vi "PathPlanner_PathFinder_DoReset.vi"   [LabVIEW 2019]
uses:
  PathPlannerLib24/VI/PathPlanner_GridPosition_Get.vi
  PathPlannerLib24/VI/PathPlanner_PathFinder_Heuristic.vi
  PathPlannerLib24/VI/PathPlanner_PathFinder_Globals.vi
  PathPlannerLib24/PathPlanner24.lvlib
types:
  T1 = typedef "PathPlanner24.lvlib/PathPlannerFinderGridPosition.ctl" = cluster{"X":i32, "Y":i32}
  T2 = typedef "PathPlanner24.lvlib/PathPlannerFinderDoublePair.ctl" = cluster{"A":dbl, "B":dbl}
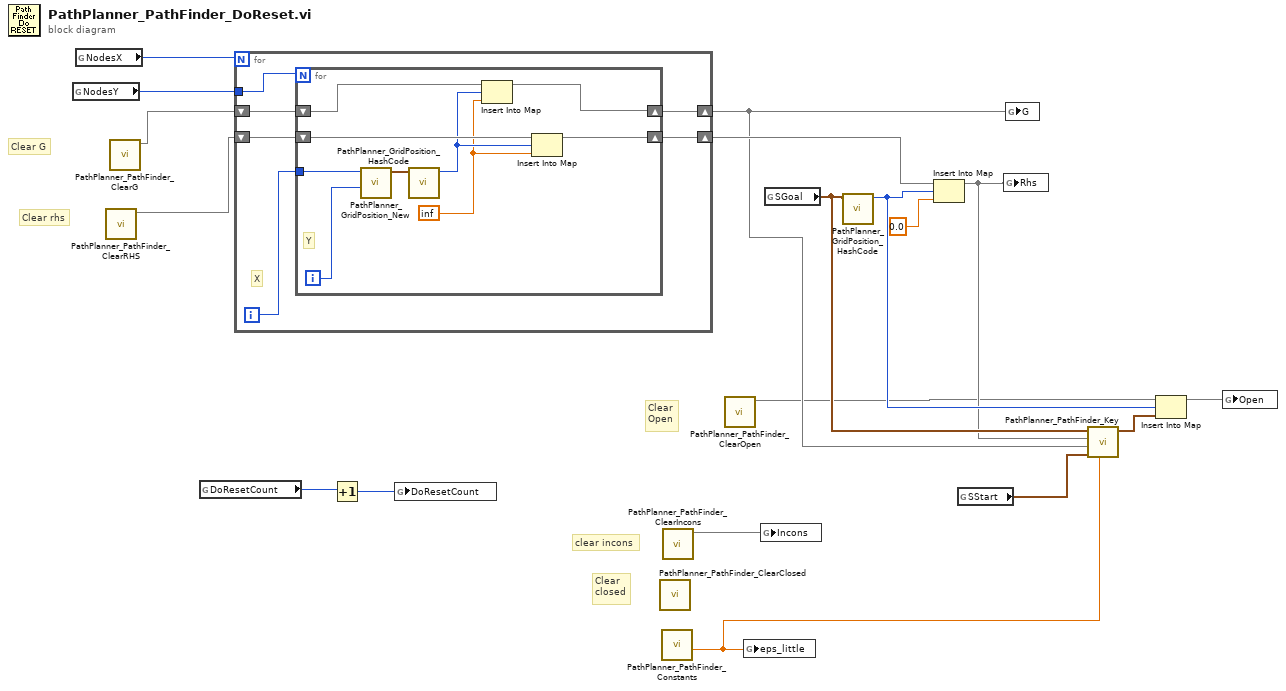
[diagram p0: block diagram]
diagram:
  # "Clear\nOpen"
  # "Clear \nclosed"
  # "clear incons"
  # "Clear rhs"
  # "Clear G"
  n1 = global read "PathPlanner_PathFinder_Globals.vi" "NodesY"() -> (w17:i32)
  n2 = global read "PathPlanner_PathFinder_Globals.vi" "NodesX"() -> (w18:i32)
  n3 = call "PathPlanner_PathFinder_ClearRHS.vi"() -> ("Rhs"=w15:map{i32, dbl})  [unwired: 11 in]
  n4 = call "PathPlanner_PathFinder_ClearG.vi"() -> ("G"=w16:map{i32, dbl})  [unwired: 11 in]
  n5 = global read "PathPlanner_PathFinder_Globals.vi" "DoResetCount"() -> (w3:i64)
  n6 = for {
    N: w18 -> [_]
    tunnel: w17 -> [w24]
    shift-right: [w20] -> w7
    shift-left: w16 -> [w23]
    shift-right: [w19] -> w14
    shift-left: w15 -> [w21]
    i -> [w22]
    # "X"
    n7 = for {
      N: w24 -> [_]
      shift-right: [w26] -> w20
      shift-left: w23 -> [w33]
      tunnel: w22 -> [w32]
      shift-right: [w25] -> w19
      shift-left: w21 -> [w29]
      i -> [w31]
      w27 = inf
      # "Y"
      n8 = call "PathPlanner_GridPosition_New.vi"("Int Y"=w31, "Int X"=w32) -> ("GridPosition"=w30:T1)  [unwired: 9 in]
      n9 = call "PathPlanner_GridPosition_HashCode.vi"("GridPosition"=w30) -> ("HashCode"=w28:i32)  [unwired: 10 in]
      n10 = Insert Into Map(map in=w33, key=w28, value=w27) -> (map out=w26:map{i32, dbl})  [unwired: 2 out]
      n11 = Insert Into Map(map in=w29, key=w28, value=w27) -> (map out=w25:map{i32, dbl})  [unwired: 2 out]
    }
  }
  n12 = Increment(x=w3) -> (x+1=w2:i64)
  n13 = global write "PathPlanner_PathFinder_Globals.vi" "DoResetCount"(w2) -> ()
  n14 = call "PathPlanner_PathFinder_ClearClosed.vi"() -> ()  [unwired: 11 in, 1 out]
  n15 = call "PathPlanner_PathFinder_Constants.vi"() -> ("EPS"=w1:dbl)  [unwired: 9 in, 2 out]
  n16 = call "PathPlanner_PathFinder_ClearIncons.vi"() -> ("Incons"=w4:map{i32, T2})  [unwired: 11 in]
  n17 = call "PathPlanner_PathFinder_ClearOpen.vi"() -> ("Open"=w5:map{i32, T2})  [unwired: 11 in]
  n18 = global write "PathPlanner_PathFinder_Globals.vi" "eps_little"(w1) -> ()
  n19 = global write "PathPlanner_PathFinder_Globals.vi" "Incons"(w4) -> ()
  n20 = global read "PathPlanner_PathFinder_Globals.vi" "SGoal"() -> (w9:T1)
  n21 = call "PathPlanner_GridPosition_HashCode.vi"("GridPosition"=w9) -> ("HashCode"=w11:i32)  [unwired: 10 in]
  n22 = Insert Into Map(map in=w14, key=w11, value=0.0) -> (map out=w8:map{i32, dbl})  [unwired: 2 out]
  n23 = global read "PathPlanner_PathFinder_Globals.vi" "SStart"() -> (w6:T1)
  n24 = global write "PathPlanner_PathFinder_Globals.vi" "Rhs"(w8) -> ()
  n25 = global write "PathPlanner_PathFinder_Globals.vi" "G"(w7) -> ()
  n26 = call "PathPlanner_PathFinder_Key.vi"("eps_little"=w1, "Sstart"=w6, "G"=w7, "RHS"=w8, "S"=w9) -> ("DoublePair"=w10:T2)  [unwired: 6 in]
  n27 = Insert Into Map(map in=w5, key=w11, value=w10) -> (map out=w12:map{i32, T2})  [unwired: 2 out]
  n28 = global write "PathPlanner_PathFinder_Globals.vi" "Open"(w12) -> ()
